vi "Select Object.vi"(10 "Coords":T12, 11 "Core Data in":T10) -> (2 "Object":T1 {"Triangles"."Vertex 3"."UV"."v" min=0 max=1 step=0.1; "Triangles"."Vertex 3"."UV"."u" min=0 max=1 step=0.1; "Triangles"."Vertex 2"."UV"."v" min=0 max=1 step=0.1; "Triangles"."Vertex 2"."UV"."u" min=0 max=1 step=0.1; "Triangles"."Vertex 1"."UV"."v" min=0 max=1 step=0.1; "Triangles"."Vertex 1"."UV"."u" min=0 max=1 step=0.1}, 3 "Core Data out":T10)   [LabVIEW 2020, in "Example 1.lvlib"]
uses:
  Example 1.lvlib
  Scene/Scene.lvclass
  <vilib>/Utility/miscctls.llb/LVPoint32TypeDef.ctl
  Core Data.ctl
  Graphics/Libraries/3D/Vector 3D.ctl
  Graphics/Libraries/3D/3D.lvlib
  Graphics/Libraries/3D/Transform.ctl
  Scene/Mouse Button Held.ctl
  Graphics/Libraries/3D/Object.ctl
  Graphics/Libraries/Raster/UV.ctl
  Graphics/Libraries/Raster/Raster.lvlib
  Graphics/Libraries/3D/Vertex.ctl
  Graphics/Libraries/3D/Triangle.ctl
  Graphics/Libraries/Raster/Rectangle Dimensions.ctl
  Graphics/Libraries/Raster/Texture.ctl
  Graphics/Libraries/3D/Material.ctl
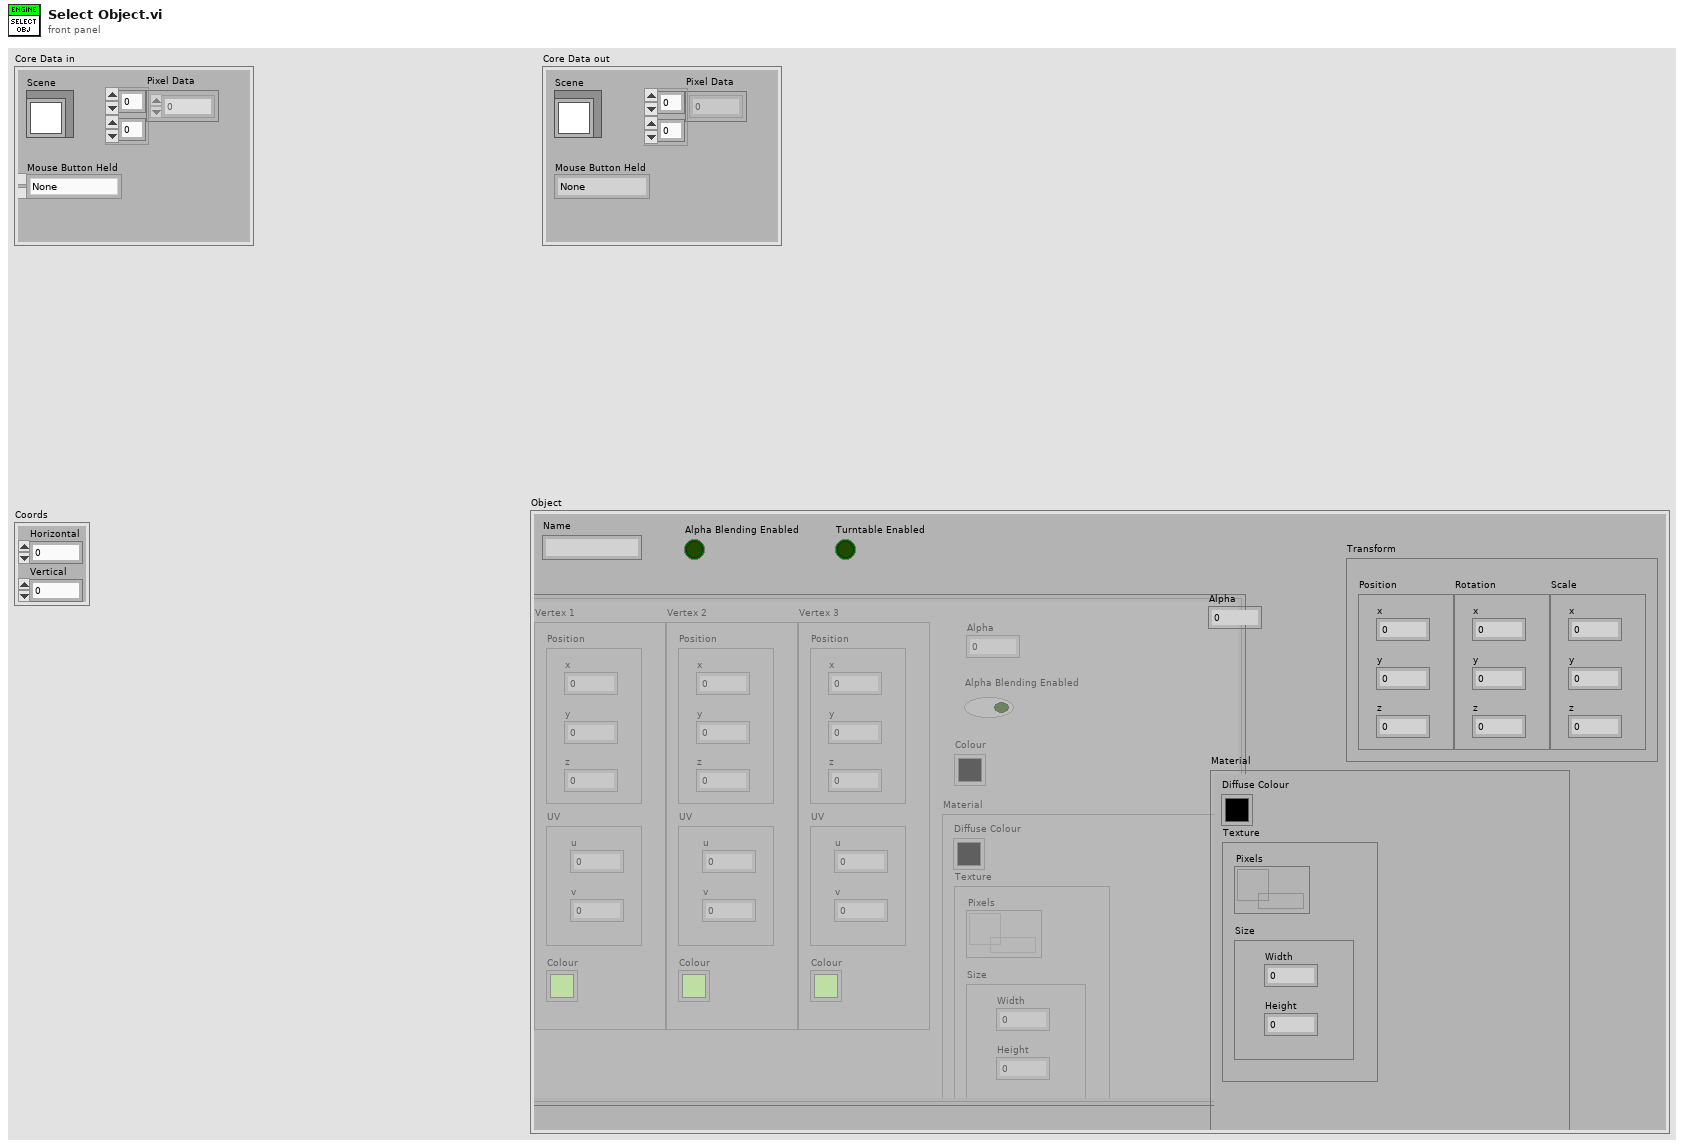
[diagram p1: front panel]
types:
  T1 = typedef "3D.lvlib/Object.ctl" = cluster{"Triangles":T2[], "Transform":T9, "Name":string, "Alpha Blending Enabled":bool, "Alpha":dbl, "Turntable Enabled":bool, "Material":T6}
  T2 = typedef "3D.lvlib/Triangle.ctl" = cluster{"Vertex 1":T3, "Vertex 2":T3, "Vertex 3":T3, "Alpha":dbl, "Alpha Blending Enabled":bool, "Colour":u32, "Material":T6}
  T3 = typedef "3D.lvlib/Vertex.ctl" = cluster{"Position":T4, "UV":T5, "Colour":u32}
  T4 = typedef "3D.lvlib/Vector 3D.ctl" = cluster{"x":sgl, "y":sgl, "z":sgl}
  T5 = typedef "Raster.lvlib/UV.ctl" = cluster{"u":sgl, "v":sgl}
  T6 = typedef "3D.lvlib/Material.ctl" = cluster{"Diffuse Colour":u32, "Texture":T7}
  T7 = typedef "Raster.lvlib/Texture.ctl" = cluster{"Pixels":refnum<data-value>, "Size":T8}
  T8 = typedef "Raster.lvlib/Rectangle Dimensions.ctl" = cluster{"Width":u32, "Height":u32}
  T9 = typedef "3D.lvlib/Transform.ctl" = cluster{"Position":T4, "Rotation":T4, "Scale":T4}
  T10 = typedef "Example 1.lvlib/Core Data.ctl" = cluster{"Pixel Data":u32[][], "Scene":refnum<class "Scene.lvclass">, "Mouse Button Held":T11}
  T11 = typedef "Scene.lvclass/Mouse Button Held.ctl" = enum16{"None", "Left", "Middle", "Right"}
  T12 = typedef "LVPoint32TypeDef.ctl" = cluster{"Horizontal":i32, "Vertical":i32}
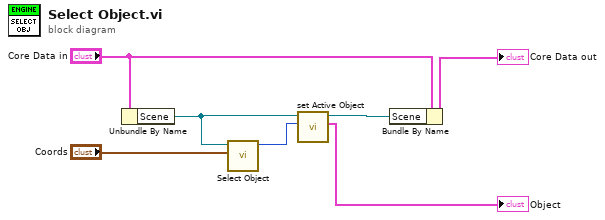
[diagram p0: block diagram]
diagram:
  n1 = Unbundle By Name("Core Data in") -> ("Scene"=w3:refnum<class "Scene.lvclass">)
  n2 = call "Select Object.vi"("Coords"="Coords", "Scene in"=w3) -> ("Active Object"=w2:i32)  [unwired: 9 in]
  n3 = call "set Active Object.vi"("Active Object"=w2, "Scene in"=w3) -> ("Object"=→"Object":T1, "Scene out"=w4:refnum<class "Scene.lvclass">)  [unwired: 8 in]
  n4 = Bundle By Name(cluster="Core Data in", "Scene"=w4) -> (→"Core Data out":T10)
